vi "HEWH Standard MW100 Data.vi"(4 "Use Emerson 5700?":bool, 6 "Use Laurel":bool, 7 "Emerson Flow Meter Data Output":T1, 8 "Error In":errorcluster, 11 "MW100 Data Cluster":T2) -> (0 "Error Out":errorcluster, 2 "Hot Side Emerson Flow Meter Data":T1, 3 "Standard MW100 Data":string[][](array[string])=[["T1", "0.000"], ["T2", "0.000"], ["T3", "0.000"], ["T4", "0.000"], ["T5", "0.000"], ["T6", "0.000"], ["T7", "0.000"], ["T8", "0.000"], ["T9", "0.000"], ["T10", "0.000"], ["TC Tree Average", "0.000"], ["TC Down", "0.000"], ["RTD IN", "0.000"], ["RTD Out", "0.000"], ["RTD Ambient", "0.000"], ["Totalized Flow (Linear Link) - Calculated (Gallons)", "0.000"], ["Flow Rate (Linear Link) - Calculated (GPM)", "0.000"], ["Pressure - HI1", "0.000"], ["Pressure - HI2", "0.000"], ["Pressure - LOW", "0.000"], ["Pressure - PIN", "0.000"]])   [LabVIEW 2016]
uses:
  Type Definitions/HEWH MW100 Data Cluster.ctl
  Drivers/Emerson 5700 Transmitter/Type Definitions/Emerson 5700 Data.ctl
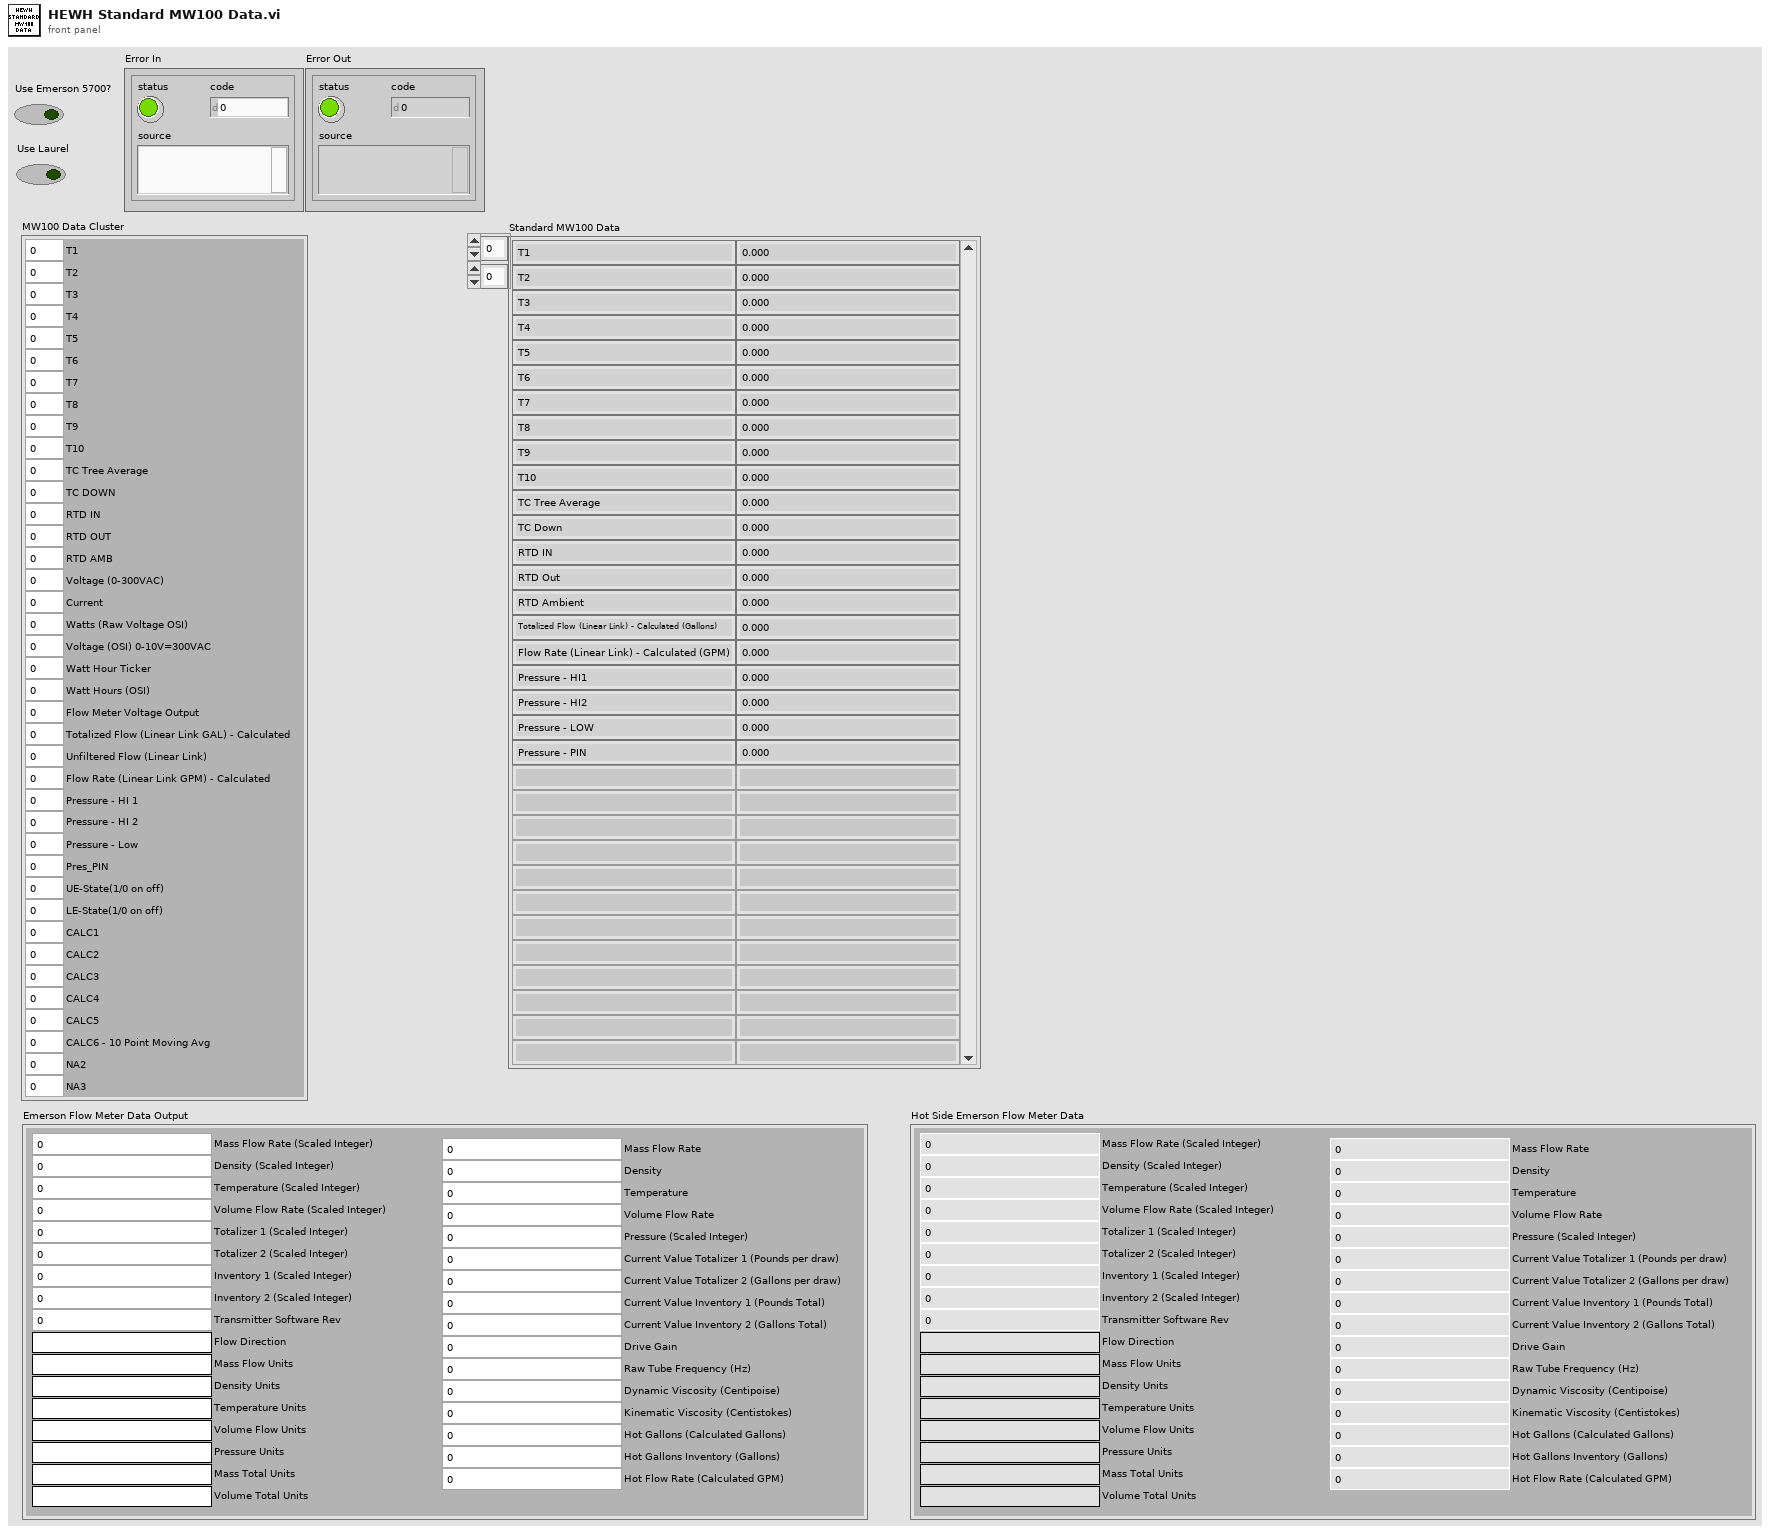
[diagram p1: front panel]
types:
  T1 = typedef "Emerson 5700 Data.ctl" = cluster{"Mass Flow Rate (Scaled Integer)":u16, "Density (Scaled Integer)":u16, "Temperature (Scaled Integer)":u16, "Volume Flow Rate (Scaled Integer)":u16, "Totalizer 1 (Scaled Integer)":u16, "Totalizer 2 (Scaled Integer)":u16, "Transmitter Software Rev":u16, "Flow Direction":string, "Mass Flow Units":string, "Density Units":string, "Temperature Units":string, "Volume Flow Units":string, "Pressure Units":string, "Mass Total Units":string, "Volume Total Units":string, "Inventory 1 (Scaled Integer)":u16, "Inventory 2 (Scaled Integer)":u16, "Mass Flow Rate":dbl, "Density":dbl, "Temperature":dbl, "Volume Flow Rate":dbl, "Pressure (Scaled Integer)":u16, "Current Value Totalizer 1 (Pounds per draw)":dbl, "Current Value Totalizer 2 (Gallons per draw)":dbl, "Current Value Inventory 1 (Pounds Total)":dbl, "Current Value Inventory 2 (Gallons Total)":dbl, "Drive Gain":dbl, "Raw Tube Frequency (Hz)":dbl, "Dynamic Viscosity (Centipoise)":dbl, "Kinematic Viscosity (Centistokes)":dbl, "Hot Gallons (Calculated Gallons)":dbl, "Hot Flow Rate (Calculated GPM)":dbl, "Hot Gallons Inventory (Gallons)":dbl}
  T2 = typedef "HEWH MW100 Data Cluster.ctl" = cluster{"T1":dbl, "T2":dbl, "T3":dbl, "T4":dbl, "T5":dbl, "T6":dbl, "T7":dbl, "T8":dbl, "T9":dbl, "T10":dbl, "TC Tree Average":dbl, "TC DOWN":dbl, "RTD IN":dbl, "RTD OUT":dbl, "RTD AMB":dbl, "Voltage (0-300VAC)":dbl, "Current":dbl, "Watts (Raw Voltage OSI)":dbl, "Voltage (OSI) 0-10V=300VAC":dbl, "Watt Hour Ticker":dbl, "Watt Hours (OSI)":dbl, "Flow Meter Voltage Output":dbl, "Totalized Flow (Linear Link GAL) - Calculated":dbl, "Unfiltered Flow (Linear Link)":dbl, "Flow Rate (Linear Link GPM) - Calculated":dbl, "Pressure - HI 1":dbl, "Pressure - HI 2":dbl, "Pressure - Low":dbl, "Pres_PIN":dbl, "UE-State(1/0 on off)":dbl, "LE-State(1/0 on off)":dbl, "CALC1":dbl, "CALC2":dbl, "CALC3":dbl, "CALC4":dbl, "CALC5":dbl, "CALC6 - 10 Point Moving Avg":dbl, "NA2":dbl, "NA3":dbl}
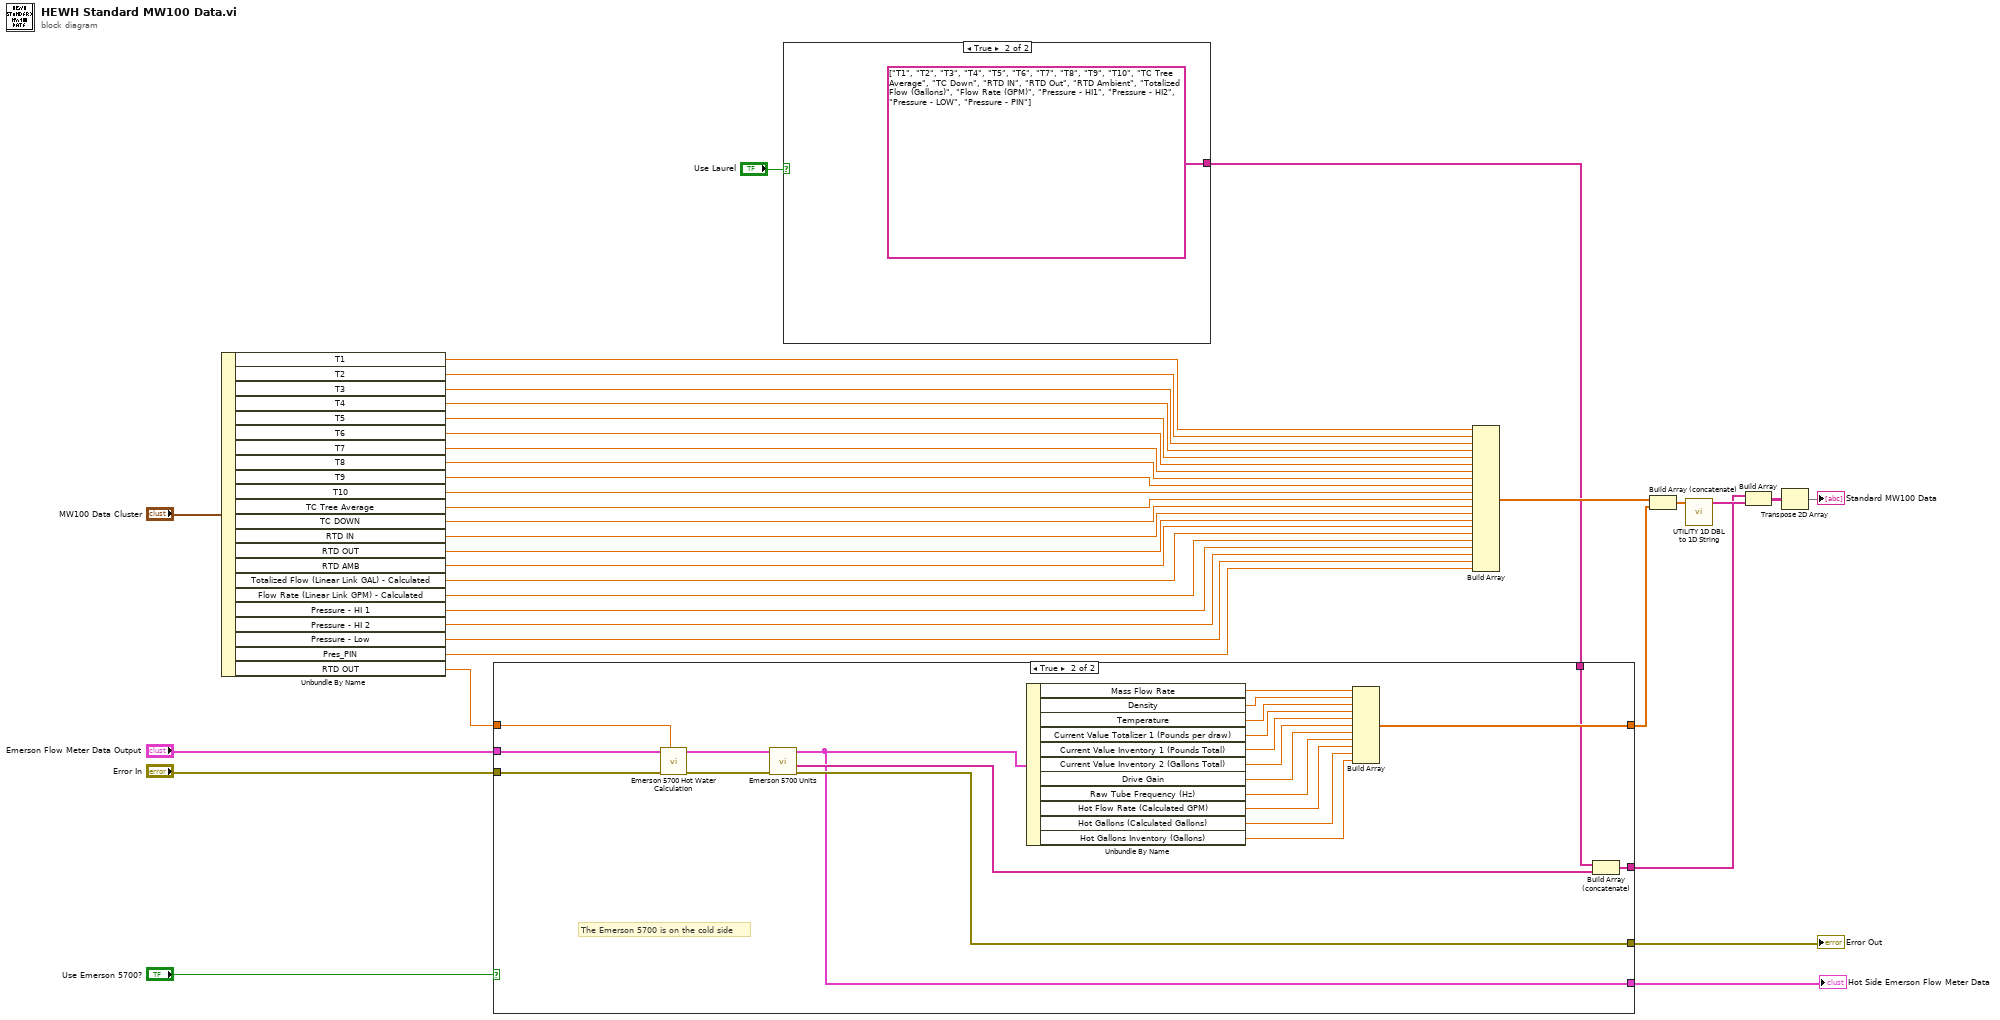
[diagram p0: block diagram]
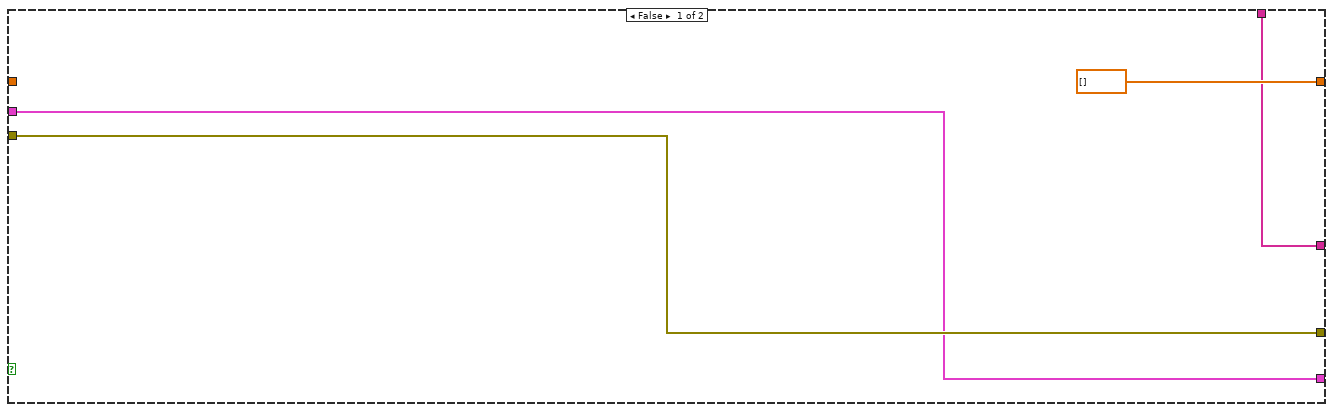
[diagram p2: hidden frame]
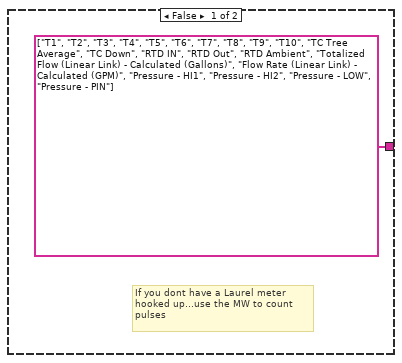
[diagram p3: hidden frame]
diagram:
  n1 = Unbundle By Name("MW100 Data Cluster") -> ("T1"=w19:dbl, "T2"=w20:dbl, "T3"=w21:dbl, "T4"=w22:dbl, "T5"=w23:dbl, "T6"=w24:dbl, "T7"=w25:dbl, "T8"=w26:dbl, "T9"=w27:dbl, "T10"=w28:dbl, "TC Tree Average"=w29:dbl, "TC DOWN"=w30:dbl, "RTD IN"=w31:dbl, "RTD OUT"=w32:dbl, "RTD AMB"=w33:dbl, "Totalized Flow (Linear Link GAL) - Calculated"=w13:dbl, "Flow Rate (Linear Link GPM) - Calculated"=w12:dbl, "Pressure - HI 1"=w34:dbl, "Pressure - HI 2"=w35:dbl, "Pressure - Low"=w36:dbl, "Pres_PIN"=w37:dbl, "RTD OUT"=w5:dbl)
  n2 = case shown="True" "Use Laurel" {
    tunnel: [string[] ["T1", "T2", "T3", "T4", "T5", "T6", "T7", "T8", "T9", "T10", "TC Tree Average", "TC Down", "RTD IN", "RTD Out", "RTD Ambient", "Totalized Flow (Linear Link) - Calculated (Gallons)", "Flow Rate (Linear Link) - Calculated (GPM)", "Pressure - HI1", "Pressure - HI2", "Pressure - LOW", "Pressure - PIN"] ("output array") string[] ["T1", "T2", "T3", "T4", "T5", "T6", "T7", "T8", "T9", "T10", "TC Tree Average", "TC Down", "RTD IN", "RTD Out", "RTD Ambient", "Totalized Flow (Gallons)", "Flow Rate (GPM)", "Pressure - HI1", "Pressure - HI2", "Pressure - LOW", "Pressure - PIN"] ("output array")] -> w7
    frame False {
      # "If you dont have a Laurel meter\nhooked up...use the MW to count\npulses"
    }
    frame True {
    }
  }
  n3 = case shown="True" "Use Emerson 5700?" {
    tunnel: [dbl[] [] w57] -> w9
    tunnel: w7 -> [w42 w56]
    tunnel: [w42 w55] -> w6
    tunnel: w5 -> [_ w50]
    tunnel: "Error In" -> [w41 w51]
    tunnel: [w41 w47] -> w3
    tunnel: [w40 w45] -> w2
    tunnel: "Emerson Flow Meter Data Output" -> [w40 w44]
    frame False {
    }
    frame True {
      # "The Emerson 5700 is on the cold side"
      n4 = call "Emerson 5700 Hot Water Calculation.vi"("RTD Out (°F)"=w50, "Error In"=w51, "Emerson Flow Meter Data Output"=w44) -> ("Error Out"=w49:errorcluster, "Emerson Flow Meter Data Output 2"=w48:T1)  [unwired: 7 in]
      n5 = call "Emerson 5700 Units.vi"("Error In"=w49, "Emerson Flow Meter Data Input"=w48) -> ("Error Out"=w47:errorcluster, "Basic Units"=w46:string[], "Emerson Flow Meter Data Output"=w45:T1)  [unwired: 6 in, 1 out]
      n6 = Unbundle By Name(w45) -> ("Mass Flow Rate"=w65:dbl, "Density"=w64:dbl, "Temperature"=w63:dbl, "Current Value Totalizer 1 (Pounds per draw)"=w62:dbl, "Current Value Inventory 1 (Pounds Total)"=w61:dbl, "Current Value Inventory 2 (Gallons Total)"=w60:dbl, "Drive Gain"=w59:dbl, "Raw Tube Frequency (Hz)"=w58:dbl, "Hot Flow Rate (Calculated GPM)"=w54:dbl, "Hot Gallons (Calculated Gallons)"=w53:dbl, "Hot Gallons Inventory (Gallons)"=w52:dbl)
      n7 = Build Array(w65, w64, w63, w62, w61, w60, w59, w58, w54, w53, w52) -> (w57:dbl[])
      n8 = Build Array (concatenate)(w56, w46) -> (w55:string[])
    }
  }
  "Error Out" <- w3
  "Hot Side Emerson Flow Meter Data" <- w2
  n9 = Build Array(w19, w20, w21, w22, w23, w24, w25, w26, w27, w28, w29, w30, w31, w32, w33, w13, w12, w34, w35, w36, w37) -> (w10:dbl[])
  n10 = Build Array (concatenate)(w10, w9) -> (w8:dbl[])
  n11 = call "UTILITY 1D DBL to 1D String.vi"("1D DBL"=w8) -> ("1D String"=w17:string[])  [unwired: 10 in]
  n12 = Build Array(w6, w17) -> (w18:string[][])
  n13 = Transpose 2D Array(2D array=w18) -> (transposed array=→"Standard MW100 Data":string[][])
